vi "Celsius to Fahrenheit.vi"() -> ()   [LabVIEW 2026]
panel:
  in  "Celsius":dbl(slide) scale=0.0..10.0
  out "Fahrenheit":dbl(slide) scale=0.0..100.0
  out "Fahrenheit":dbl
  in  "Celsius":dbl
  # "Version 1: Standard Numeric Inputs (Basic Equation Setup)"
  # "Version 2: Upgraded Application Using Graphical Sliders and Interactive Temperature Indicators"
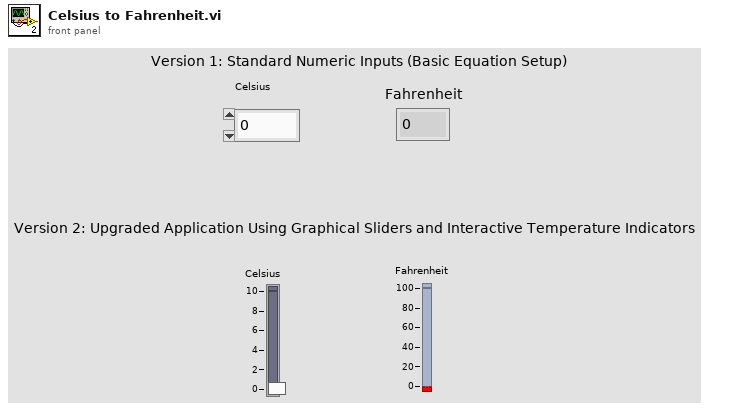
[diagram p1: front panel]
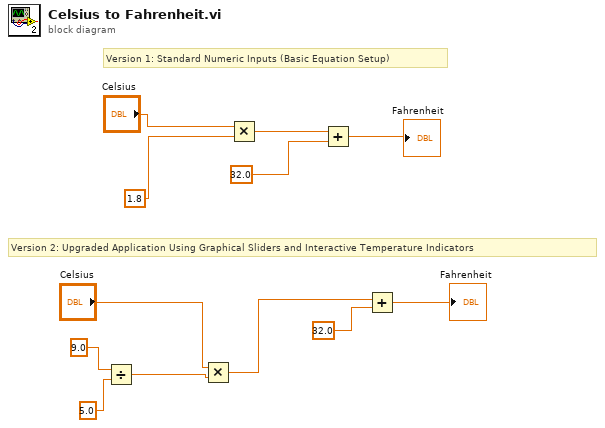
[diagram p0: block diagram]
diagram:
  # "Version 1: Standard Numeric Inputs (Basic Equation Setup)"
  # "Version 2: Upgraded Application Using Graphical Sliders and Interactive Temperature Indicators"
  n1 = Divide(x=9.0, y=5.0) -> (x/y=w5:dbl)
  n2 = Multiply(x="Celsius", y=w5) -> (x*y=w3:dbl)
  n3 = Multiply(x="Celsius", y=1.8 ("x*y")) -> (x*y=w10:dbl)
  n4 = Add(x=w10, y=32.0) -> (x+y=→"Fahrenheit":dbl)
  n5 = Add(x=w3, y=32.0) -> (x+y=→"Fahrenheit":dbl)
